vi "Feed.vi"(0 "LINX Resource":T1={"IO"=enum."Remote", "Interface"=enum."Serial", "LINX Device Config"={"Interface"=enum."Serial", "COM Port"="COM13", "TCP Configuration"={"IP Address"="", "Port"=0}, "Device Family"=1, "Device ID"=1, "Device Name"="myRIO-1900", "TCP Ref"=refnum, "Channels"={"DI"=[0, 1, 2, 3, 4, 5, 6, 7, 8, 9, 10, 11, 12, 13, 14, 15, 16, 17, 18, 19, 20, 21, 22, 23, 24, 25, 26, 27, 28, 29, 30, 31, 32, 33, 34, 35, 36, 37, 38, 39, 40, 41, 42, 43, 44, 45, 46], "DO"=[0, 1, 2, 3, 4, 5, 6, 7, 8, 9, 10, 11, 12, 13, 14, 15, 16, 17, 18, 19, 20, 21, 22, 23, 24, 25, 26, 27, 28, 29, 30, 31, 32, 33, 34, 35, 36, 37, 38, 39, 40, 41, 42, 43, 44, 45, 46], "AI"=[0, 1, 2, 3, 4, 5, 6, 7, 8, 9, 10, 11], "AO"=[], "PWM"=[3, 5, 6, 9, 10], "QE"=[], "UART"=[0, 1], "I2C 2"=[0], "SPI"=[0], "CAN"=[], "Servo"=[], "AI Ref (V)"=0.0, "AI Resolution (Bits)"=0, "AO Ref (V)"=0.0, "AO Resolution (Bits)"=0}}}, 5 "Channel":u32, 7 "Ring":u16, 9 "Feed Cycles":i32, 11 "All Rings":bool, 12 "error in (no error)":errorcluster) -> (4 "LINX Resource out":T1, 15 "error out":errorcluster)   [LabVIEW 2018]
uses:
  <vilib>/MakerHub/LINX/Private/Type Defs/LINX Ref.ctl
  <vilib>/MakerHub/LINX/Private/Type Defs/Platform.ctl
  <vilib>/MakerHub/LINX/Private/Type Defs/Interface.ctl
  <vilib>/MakerHub/LINX/Private/Device/Type Defs/LINX Device Config.ctl
  <vilib>/MakerHub/LINX/Private/Device/Type Defs/TCP Config.ctl
  <vilib>/MakerHub/LINX/Private/Device/Type Defs/Channels.ctl
  <vilib>/MakerHub/LINX/Public/Peripherals/Digital/Digital Write N Chans.vi
  <vilib>/MakerHub/LINX/Private/Local IO/LinxDigitalWrite.vi
  <vilib>/MakerHub/LINX/Public/Utilities/Check Channel.vi
  <vilib>/MakerHub/LINX/Private/Utilties/Generate Error.vi
  <vilib>/MakerHub/LINX/LMH-LINX.lvlib
  <vilib>/MakerHub/LINX/Private/Device/Device.lvlib
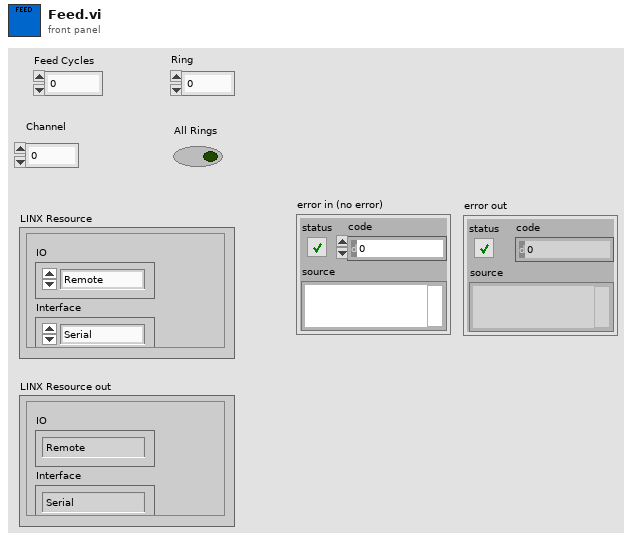
[diagram p1: front panel]
types:
  T1 = typedef "LMH-LINX.lvlib/LINX Ref.ctl" = cluster{"IO":T2, "Interface":T3, "LINX Device Config":T4}
  T2 = typedef "LMH-LINX.lvlib/Platform.ctl" = enum16{"Remote", "Local"}
  T3 = typedef "LMH-LINX.lvlib/Interface.ctl" = enum16{"Serial", "TCP"}
  T4 = typedef "LMH-LINX.lvlib/Device.lvlib/LINX Device Config.ctl" = cluster{"Interface":T3, "COM Port":refnum<visa-resource-name>, "TCP Configuration":T5, "Device Family":u8, "Device ID":u8, "Device Name":string, "TCP Ref":refnum<k5>, "Channels":T6}
  T5 = typedef "LMH-LINX.lvlib/Device.lvlib/TCP Config.ctl" = cluster{"IP Address":string, "Port":u16}
  T6 = typedef "LMH-LINX.lvlib/Channels.ctl" = cluster{"DI":u8[], "DO":u8[], "AI":u8[], "AO":u8[], "PWM":u8[], "QE":u8[], "UART":u8[], "I2C 2":u8[], "SPI":u8[], "CAN":u8[], "Servo":u8[], "AI Ref (V)":dbl, "AI Resolution (Bits)":u8, "AO Ref (V)":dbl, "AO Resolution (Bits)":u8}
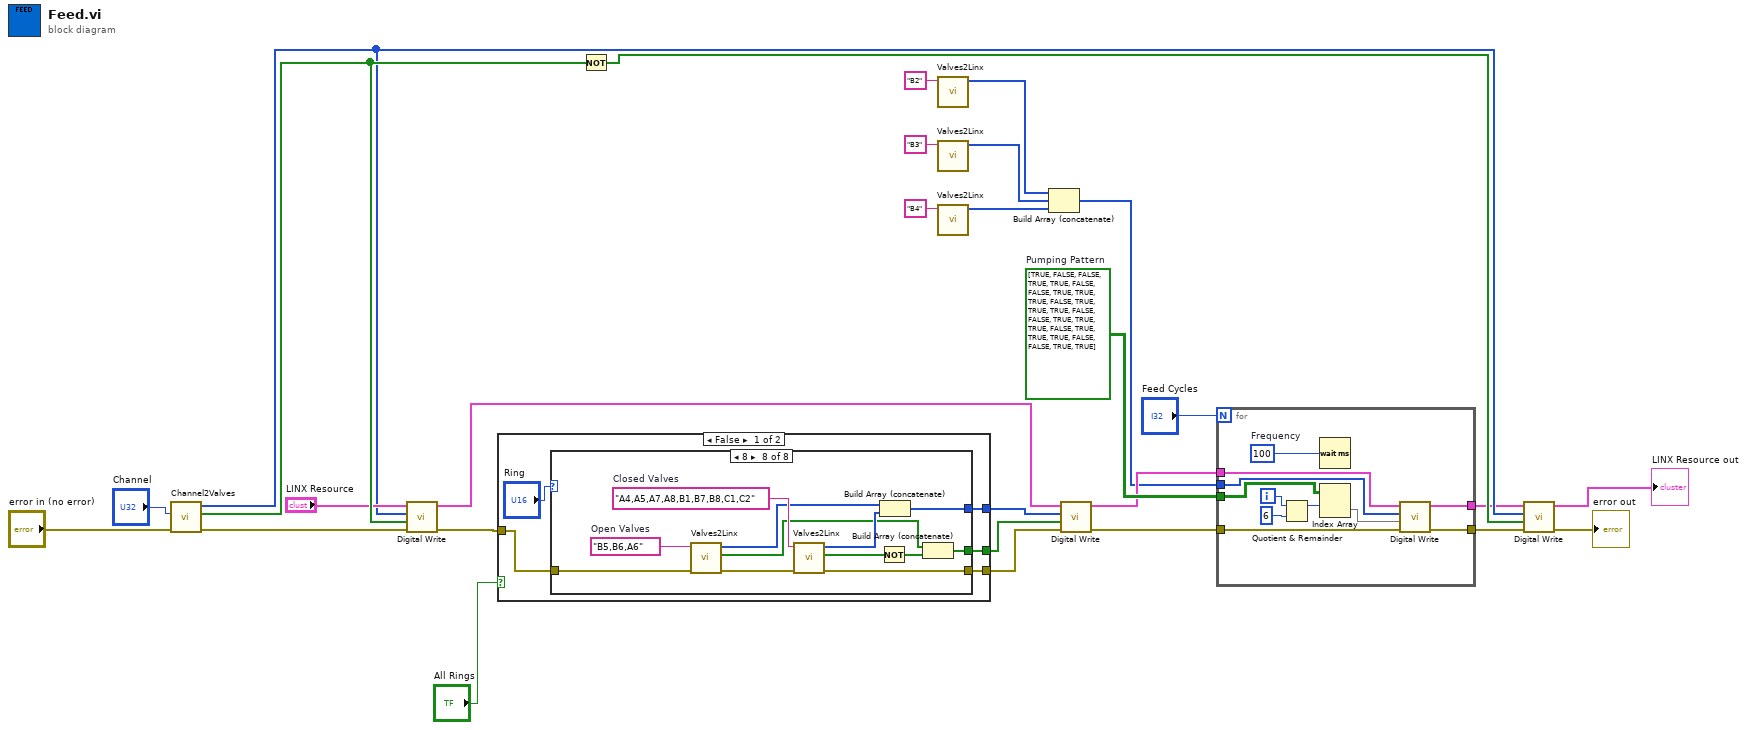
[diagram p0: block diagram]
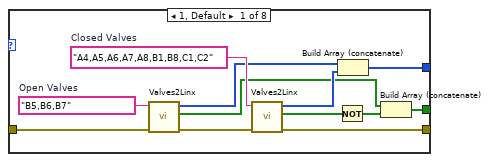
[diagram p2: hidden frame]
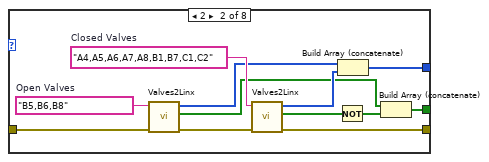
[diagram p3: hidden frame]
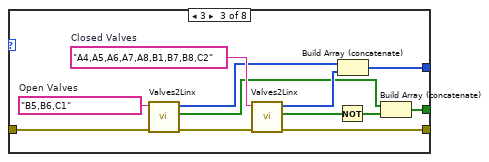
[diagram p4: hidden frame]
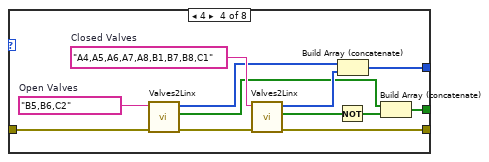
[diagram p5: hidden frame]
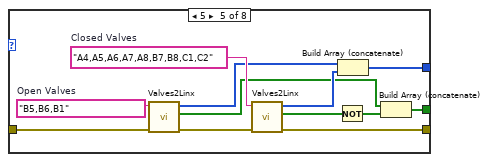
[diagram p6: hidden frame]
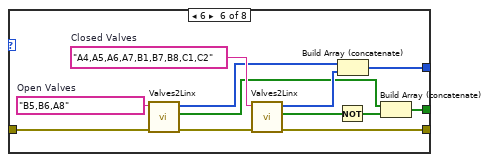
[diagram p7: hidden frame]
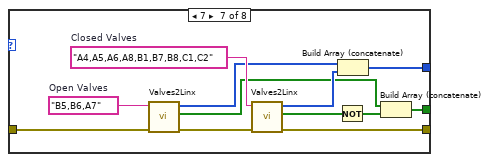
[diagram p8: hidden frame]
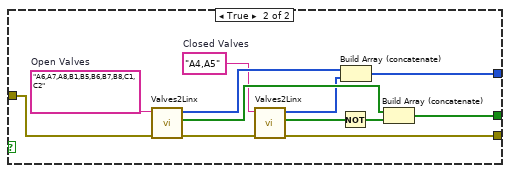
[diagram p9: hidden frame]
diagram:
  w16 = bool[][] [[TRUE, FALSE, FALSE], [TRUE, TRUE, FALSE], [FALSE, TRUE, TRUE], [TRUE, FALSE, TRUE], [TRUE, TRUE, FALSE], [FALSE, TRUE, TRUE], [TRUE, FALSE, TRUE], [TRUE, TRUE, FALSE], [FALSE, TRUE, TRUE]]  # Pumping Pattern
  n1 = call "Channel2Valves.vi"("Channel"="Channel", "error in (no error)"="error in (no error)") -> ("Valve Nums"=w18:i32[], "Valve State"=w25:bool[], "error out"=w27:errorcluster)  [unwired: 6 in]
  n2 = call-poly <vilib>:"Digital Write.vi"("Error In"=w27, "Values"=w25, "DO Channels"=w18, "LINX Resource"="LINX Resource") -> ("Error Out"=w15:errorcluster, "LINX Resource"=w11:T1)  [unwired: 6 in]
  n3 = case shown="False" "All Rings" {
    tunnel: w15 -> [w32 w134]
    tunnel: [w31 w132] -> w14
    tunnel: [w30 w133] -> w13
    tunnel: [w29 w131] -> w12
    frame False {
      n4 = case shown="8" "Ring" {
        tunnel: w32 -> [w37 w49 w61 w73 w85 w97 w109 w121]
        tunnel: [w36 w48 w60 w72 w84 w96 w108 w120] -> w31
        tunnel: [w35 w47 w59 w71 w83 w95 w107 w119] -> w30
        tunnel: [w34 w46 w58 w70 w82 w94 w106 w118] -> w29
        frame 1, Default {
          w44 = "A4,A5,A6,A7,A8,B1,B8,C1,C2"  # Closed Valves
          w45 = "B5,B6,B7"  # Open Valves
          n5 = call "Valves2Linx.vi"("error in (no error)"=w37, "Valve (A1-C8),\n comma separated"=w45) -> ("error out"=w38:errorcluster, "Array"=w40:bool[], "Array 2"=w41:i32[])  [unwired: 7 in]
          n6 = call "Valves2Linx.vi"("error in (no error)"=w38, "Valve (A1-C8),\n comma separated"=w44) -> ("error out"=w36:errorcluster, "Array"=w43:bool[], "Array 2"=w42:i32[])  [unwired: 7 in]
          n7 = Not(x=w43) -> (.not. x?=w39:bool[])
          n8 = Build Array (concatenate)(w41, w42) -> (w34:i32[])
          n9 = Build Array (concatenate)(w40, w39) -> (w35:bool[])
        }
        frame 2 {
          w56 = "A4,A5,A6,A7,A8,B1,B7,C1,C2"  # Closed Valves
          w57 = "B5,B6,B8"  # Open Valves
          n10 = call "Valves2Linx.vi"("error in (no error)"=w49, "Valve (A1-C8),\n comma separated"=w57) -> ("error out"=w50:errorcluster, "Array"=w52:bool[], "Array 2"=w53:i32[])  [unwired: 7 in]
          n11 = call "Valves2Linx.vi"("error in (no error)"=w50, "Valve (A1-C8),\n comma separated"=w56) -> ("error out"=w48:errorcluster, "Array"=w55:bool[], "Array 2"=w54:i32[])  [unwired: 7 in]
          n12 = Not(x=w55) -> (.not. x?=w51:bool[])
          n13 = Build Array (concatenate)(w53, w54) -> (w46:i32[])
          n14 = Build Array (concatenate)(w52, w51) -> (w47:bool[])
        }
        frame 3 {
          w68 = "A4,A5,A6,A7,A8,B1,B7,B8,C2"  # Closed Valves
          w69 = "B5,B6,C1"  # Open Valves
          n15 = call "Valves2Linx.vi"("error in (no error)"=w61, "Valve (A1-C8),\n comma separated"=w69) -> ("error out"=w62:errorcluster, "Array"=w64:bool[], "Array 2"=w65:i32[])  [unwired: 7 in]
          n16 = call "Valves2Linx.vi"("error in (no error)"=w62, "Valve (A1-C8),\n comma separated"=w68) -> ("error out"=w60:errorcluster, "Array"=w67:bool[], "Array 2"=w66:i32[])  [unwired: 7 in]
          n17 = Not(x=w67) -> (.not. x?=w63:bool[])
          n18 = Build Array (concatenate)(w65, w66) -> (w58:i32[])
          n19 = Build Array (concatenate)(w64, w63) -> (w59:bool[])
        }
        frame 4 {
          w80 = "A4,A5,A6,A7,A8,B1,B7,B8,C1"  # Closed Valves
          w81 = "B5,B6,C2"  # Open Valves
          n20 = call "Valves2Linx.vi"("error in (no error)"=w73, "Valve (A1-C8),\n comma separated"=w81) -> ("error out"=w74:errorcluster, "Array"=w76:bool[], "Array 2"=w77:i32[])  [unwired: 7 in]
          n21 = call "Valves2Linx.vi"("error in (no error)"=w74, "Valve (A1-C8),\n comma separated"=w80) -> ("error out"=w72:errorcluster, "Array"=w79:bool[], "Array 2"=w78:i32[])  [unwired: 7 in]
          n22 = Not(x=w79) -> (.not. x?=w75:bool[])
          n23 = Build Array (concatenate)(w77, w78) -> (w70:i32[])
          n24 = Build Array (concatenate)(w76, w75) -> (w71:bool[])
        }
        frame 5 {
          w92 = "A4,A5,A6,A7,A8,B7,B8,C1,C2"  # Closed Valves
          w93 = "B5,B6,B1"  # Open Valves
          n25 = call "Valves2Linx.vi"("error in (no error)"=w85, "Valve (A1-C8),\n comma separated"=w93) -> ("error out"=w86:errorcluster, "Array"=w88:bool[], "Array 2"=w89:i32[])  [unwired: 7 in]
          n26 = call "Valves2Linx.vi"("error in (no error)"=w86, "Valve (A1-C8),\n comma separated"=w92) -> ("error out"=w84:errorcluster, "Array"=w91:bool[], "Array 2"=w90:i32[])  [unwired: 7 in]
          n27 = Not(x=w91) -> (.not. x?=w87:bool[])
          n28 = Build Array (concatenate)(w89, w90) -> (w82:i32[])
          n29 = Build Array (concatenate)(w88, w87) -> (w83:bool[])
        }
        frame 6 {
          w104 = "A4,A5,A6,A7,B1,B7,B8,C1,C2"  # Closed Valves
          w105 = "B5,B6,A8"  # Open Valves
          n30 = call "Valves2Linx.vi"("error in (no error)"=w97, "Valve (A1-C8),\n comma separated"=w105) -> ("error out"=w98:errorcluster, "Array"=w100:bool[], "Array 2"=w101:i32[])  [unwired: 7 in]
          n31 = call "Valves2Linx.vi"("error in (no error)"=w98, "Valve (A1-C8),\n comma separated"=w104) -> ("error out"=w96:errorcluster, "Array"=w103:bool[], "Array 2"=w102:i32[])  [unwired: 7 in]
          n32 = Not(x=w103) -> (.not. x?=w99:bool[])
          n33 = Build Array (concatenate)(w101, w102) -> (w94:i32[])
          n34 = Build Array (concatenate)(w100, w99) -> (w95:bool[])
        }
        frame 7 {
          w116 = "A4,A5,A6,A8,B1,B7,B8,C1,C2"  # Closed Valves
          w117 = "B5,B6,A7"  # Open Valves
          n35 = call "Valves2Linx.vi"("error in (no error)"=w109, "Valve (A1-C8),\n comma separated"=w117) -> ("error out"=w110:errorcluster, "Array"=w112:bool[], "Array 2"=w113:i32[])  [unwired: 7 in]
          n36 = call "Valves2Linx.vi"("error in (no error)"=w110, "Valve (A1-C8),\n comma separated"=w116) -> ("error out"=w108:errorcluster, "Array"=w115:bool[], "Array 2"=w114:i32[])  [unwired: 7 in]
          n37 = Not(x=w115) -> (.not. x?=w111:bool[])
          n38 = Build Array (concatenate)(w113, w114) -> (w106:i32[])
          n39 = Build Array (concatenate)(w112, w111) -> (w107:bool[])
        }
        frame 8 {
          w128 = "A4,A5,A7,A8,B1,B7,B8,C1,C2"  # Closed Valves
          w129 = "B5,B6,A6"  # Open Valves
          n40 = call "Valves2Linx.vi"("error in (no error)"=w121, "Valve (A1-C8),\n comma separated"=w129) -> ("error out"=w122:errorcluster, "Array"=w124:bool[], "Array 2"=w125:i32[])  [unwired: 7 in]
          n41 = call "Valves2Linx.vi"("error in (no error)"=w122, "Valve (A1-C8),\n comma separated"=w128) -> ("error out"=w120:errorcluster, "Array"=w127:bool[], "Array 2"=w126:i32[])  [unwired: 7 in]
          n42 = Not(x=w127) -> (.not. x?=w123:bool[])
          n43 = Build Array (concatenate)(w125, w126) -> (w118:i32[])
          n44 = Build Array (concatenate)(w124, w123) -> (w119:bool[])
        }
      }
    }
    frame True {
      w135 = "A4,A5"  # Closed Valves
      w130 = "A6,A7,A8,B1,B5,B6,B7,B8,C1,C2"  # Open Valves
      n45 = call "Valves2Linx.vi"("error in (no error)"=w134, "Valve (A1-C8),\n comma separated"=w130) -> ("error out"=w141:errorcluster, "Array"=w139:bool[], "Array 2"=w138:i32[])  [unwired: 7 in]
      n46 = call "Valves2Linx.vi"("error in (no error)"=w141, "Valve (A1-C8),\n comma separated"=w135) -> ("error out"=w132:errorcluster, "Array"=w136:bool[], "Array 2"=w137:i32[])  [unwired: 7 in]
      n47 = Not(x=w136) -> (.not. x?=w140:bool[])
      n48 = Build Array (concatenate)(w138, w137) -> (w131:i32[])
      n49 = Build Array (concatenate)(w139, w140) -> (w133:bool[])
    }
  }
  n50 = Not(x=w25) -> (.not. x?=w19:bool[])
  n51 = call "Valves2Linx.vi"("Valve (A1-C8),\n comma separated"="B2") -> ("Array 2"=w5:i32[])  [unwired: 8 in, 2 out]
  n52 = call "Valves2Linx.vi"("Valve (A1-C8),\n comma separated"="B3") -> ("Array 2"=w4:i32[])  [unwired: 8 in, 2 out]
  n53 = call "Valves2Linx.vi"("Valve (A1-C8),\n comma separated"="B4") -> ("Array 2"=w3:i32[])  [unwired: 8 in, 2 out]
  n54 = Build Array (concatenate)(w5, w4, w3) -> (w2:i32[])
  n55 = call-poly <vilib>:"Digital Write.vi"("Error In"=w14, "Values"=w13, "DO Channels"=w12, "LINX Resource"=w11) -> ("Error Out"=w9:errorcluster, "LINX Resource"=w10:T1)  [unwired: 6 in]
  n56 = for {
    N: "Feed Cycles" -> [_]
    tunnel: w9 -> [w148]
    tunnel: [w142] -> w24
    tunnel: w10 -> [w149]
    tunnel: [w143] -> w17
    tunnel: w16 -> [w146]
    tunnel: w2 -> [w147]
    i -> [w150]
    w152 = u32 100  # Frequency
    n57 = Quotient & Remainder(x=w150, y=6) -> (x-y*floor(x/y)=w144:i32)  [unwired: 1 out]
    n58 = Wait (ms)(milliseconds to wait=w152) -> ()  [unwired: 1 out]
    n59 = Index Array(array=w146, index (row)=w144) -> (element=w145:bool[])  [unwired: 1 in]
    n60 = call-poly <vilib>:"Digital Write.vi"("Error In"=w148, "Values"=w145, "DO Channels"=w147, "LINX Resource"=w149) -> ("Error Out"=w142:errorcluster, "LINX Resource"=w143:T1)  [unwired: 6 in]
  }
  n61 = call-poly <vilib>:"Digital Write.vi"("Error In"=w24, "Values"=w19, "DO Channels"=w18, "LINX Resource"=w17) -> ("Error Out"=→"error out":errorcluster, "LINX Resource"=→"LINX Resource out":T1)  [unwired: 6 in]
